vi "Cambio UM Q.vi"(10 "Q[mh3]":dbl, 11 "UM":T1) -> (3 "Q [UM]":dbl)   [LabVIEW 2019]
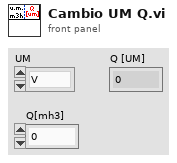
[diagram p1: front panel]
types:
  T1 = typedef "UnitàMisura.ctl" = enum16{"V", "mA", "Bar", "RPM", "m3/s", "m3/min", "m3/h", "l/s", "l/min", "in3/min", "ft3/min", "gpm", "igpm", "igph", "%", "°C", "m", "Nm", "A"}
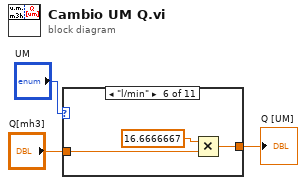
[diagram p0: block diagram]
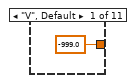
[diagram p2: hidden frame]
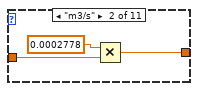
[diagram p3: hidden frame]
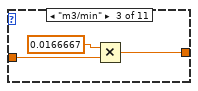
[diagram p4: hidden frame]
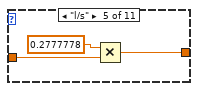
[diagram p6: hidden frame]
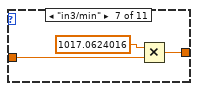
[diagram p7: hidden frame]
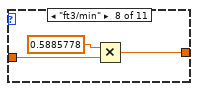
[diagram p8: hidden frame]
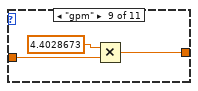
[diagram p9: hidden frame]
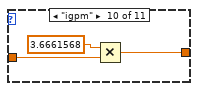
[diagram p10: hidden frame]
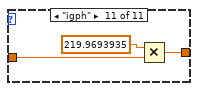
[diagram p11: hidden frame]
diagram:
  n1 = case shown="\"l/min\"" "UM" {
    tunnel: "Q[mh3]" -> [_ w7 w10 w11 w14 w17 w20 w23 w26 w29 w32]
    tunnel: [-999.0 ("mh3") w5 w9 w11 w13 w16 w19 w22 w25 w28 w31] -> w3
    frame "V", Default {
    }
    frame "m3/s" {
      n2 = Multiply(x=0.0002778, y=w7) -> (x*y=w5:dbl)
    }
    frame "m3/min" {
      n3 = Multiply(x=0.0166667, y=w10) -> (x*y=w9:dbl)
    }
    frame "m3/h" {
    }
    frame "l/s" {
      n4 = Multiply(x=0.2777778, y=w14) -> (x*y=w13:dbl)
    }
    frame "l/min" {
      n5 = Multiply(x=16.6666667, y=w17) -> (x*y=w16:dbl)
    }
    frame "in3/min" {
      n6 = Multiply(x=1017.0624016, y=w20) -> (x*y=w19:dbl)
    }
    frame "ft3/min" {
      n7 = Multiply(x=0.5885778, y=w23) -> (x*y=w22:dbl)
    }
    frame "gpm" {
      n8 = Multiply(x=4.4028673, y=w26) -> (x*y=w25:dbl)
    }
    frame "igpm" {
      n9 = Multiply(x=3.6661568, y=w29) -> (x*y=w28:dbl)
    }
    frame "igph" {
      n10 = Multiply(x=219.9693935, y=w32) -> (x*y=w31:dbl)
    }
  }
  "Q [UM]" <- w3
